vi "DIAdem Window To Top.vi"(4 "error in (no error)":errorcluster, 7 "window refnum":T1) -> (0 "error out":errorcluster)   [LabVIEW 2017]
doc: "This VI will make the window identified by the 'window refnum' the top window and activate it. If the window cannot be found, an error will be returned."
uses:
  <vilib>/ExportToExcel/Window Refnum.ctl
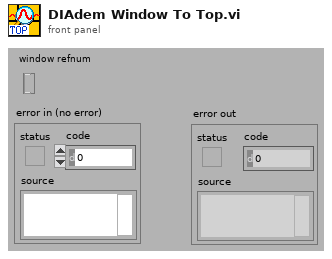
[diagram p1: front panel]
types:
  T1 = typedef "Window Refnum.ctl" = refnum<k1>
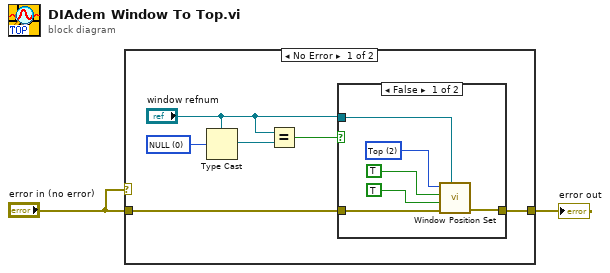
[diagram p0: block diagram]
diagram:
  n1 = case shown="No Error" "error in (no error)" {
    tunnel: "error in (no error)" -> [w3 w16]
    tunnel: [w5 w16] -> w1
    frame No Error {
      w8 = u32 0 items=["NULL"]
      n2 = Type Cast(type="window refnum", x=w8) -> (*(type *) &x=w6:T1)
      n3 = Equal?(x="window refnum", y=w6) -> (x = y?=w7:bool)
      n4 = case shown="False" w7 {
        tunnel: w3 -> [w14 w15]
        tunnel: [w13 w15] -> w5
        tunnel: "window refnum" -> [w12 _]
        frame False {
          w11 = i16 2 items=["Not Topmost", "Topmost", "Top", "Bottom"] ("window position")
          n5 = call <vilib>:"Window Position Set.vi"("window refnum"=w12, "error in (no error)"=w14, "activate error message? (T)"=TRUE ("error message? (T)"), "activate window? (T)"=TRUE ("activate? (T)"), "window position"=w11) -> ("error out"=w13:errorcluster)  [unwired: 3 in]
        }
        frame True {
        }
      }
    }
    frame Error {
    }
  }
  "error out" <- w1
